vi "drag_quantities.vi"(6 "velocity_magnitude":dbl, 7 "angle_input":i16, 9 "area":dbl, 10 "medium_density":dbl, 11 "drag-coefficient":dbl) -> (1 "drag_y_component":dbl, 2 "drag_x_component":dbl, 3 "drag_magnitude":dbl)   [LabVIEW 2018]
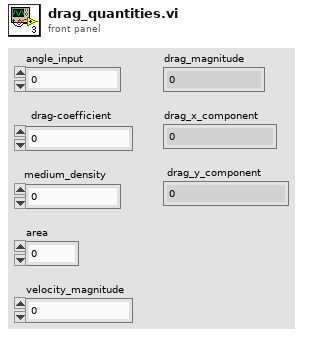
[diagram p1: front panel]
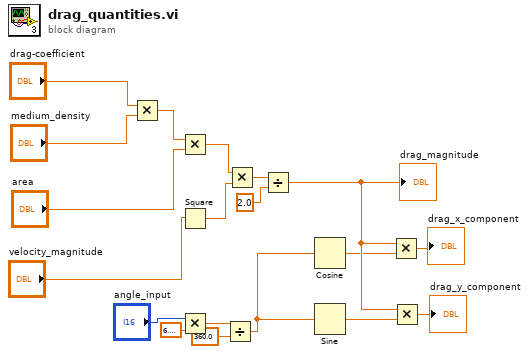
[diagram p0: block diagram]
diagram:
  n1 = Multiply(x="drag-coefficient", y="medium_density") -> (x*y=w13:dbl)
  n2 = Multiply(x=w13, y="area") -> (x*y=w15:dbl)
  n3 = Square(x="velocity_magnitude") -> (x^2=w16:dbl)
  n4 = Multiply(x="angle_input", y=6.283185307179586) -> (x*y=w3:dbl)
  n5 = Divide(x=w3, y=360.0) -> (x/y=w1:dbl)
  n6 = Multiply(x=w15, y=w16) -> (x*y=w17:dbl)
  n7 = Divide(x=w17, y=2.0) -> (x/y=w10:dbl)
  "drag_magnitude" <- w10
  n8 = Cosine(x=w1) -> (cos(x)=w9:dbl)
  n9 = Sine(x=w1) -> (sin(x)=w8:dbl)
  n10 = Multiply(x=w10, y=w9) -> (x*y=→"drag_x_component":dbl)
  n11 = Multiply(x=w10, y=w8) -> (x*y=→"drag_y_component":dbl)
